vi "HPLC software.vi"() -> ()   [LabVIEW 2014]
panel:
  out "Current Element 3":string
  in  "Baseline":bool
  in  "Lac end":dbl=6.0 format="%.2f"
  in  "Lac start":sgl=5.0 format="%.2f"
  in  "Xyl":dbl=4.0 format="%.2f"
  in  "GluXyl not important":dbl=3.0 format="%.2f"
  in  "Glu":dbl=1.0 format="%.2f"
  out "error out":errorcluster
  in  "Add 6":bool caption="Add"
  in  "Add element 6":string
  in  "Baseline 6":bool
  in  "Reset list 6":bool
  in  "Add 5":bool caption="Add"
  in  "Add element 5":string
  in  "Baseline 5":bool
  in  "Reset list 5":bool
  in  "Add 4":bool caption="Add"
  in  "Add element 4":string
  in  "Baseline 4":bool
  in  "Reset list 4":bool
  out "mean 3":dbl format="%0.2f"
  in  "Baseline 3":bool
  in  "Baseline 2":bool
  in  "Add element 2":string
  in  "Add 2":bool caption="Add"
  in  "Reset list 2":bool
  out "Glu concentration":dbl format="%.4f"
  out "?":cluster{"all rows":dbl[], "all rows":dbl[]}(graph)
  out "Xyl concentration":dbl format="%.4f"
  out "Lac concentration":dbl format="%.4f"
  in  "Glu standard area":dbl=2.0 format="%.2f"
  in  "Xyl standard area":dbl=3.0 format="%.2f"
  out "Glu area":dbl format="%.4f"
  out "Xyl area":dbl format="%.4f"
  in  "Lac standard area":dbl=4.0 format="%.2f"
  out "Lac area":dbl format="%.4f"
  in  "Reset list":bool
  in  "Add":bool
  in  "Add element 1":string
  in  "Path 1":path
  in  "Path 2":path
  in  "Path 4":path
  in  "Path 5":path
  in  "Path 6":path
  out "mean 6":dbl format="%0.2f"
  out "Device 6":cluster{dbl[], dbl[]}(graph)
  out "Current Element 6":string
  out "All samples":i32
  in  "Sample list 6":i32(listbox)
  out "Elapsed Time (s) 6":dbl
  in  "Time Target (s) 6":dbl=1.0
  out "mean 5":dbl format="%0.2f"
  out "Device 5":cluster{dbl[], dbl[]}(graph)
  out "Current Element 5":string
  out "All samples":i32
  in  "Sample list 5":i32(listbox)
  out "Elapsed Time (s) 5":dbl
  in  "Time Target (s) 5":dbl=1.0
  out "mean 4":dbl format="%0.2f"
  out "Device 4":cluster{dbl[], dbl[]}(graph)
  out "Current Element 4":string
  out "All samples":i32
  in  "Sample list 4":i32(listbox)
  out "Elapsed Time (s) 4":dbl
  in  "Time Target (s) 4":dbl=1.0
  out "JJ channel 2":cluster{dbl[], dbl[]}(graph)
  out "mean 2":dbl format="%0.2f"
  out "JJ channel 1":cluster{dbl[], dbl[]}(graph)
  out "Current Element 2":string
  out "All samples":i32
  in  "Sample list 2":i32(listbox)
  out "Elapsed Time (s) 2":dbl
  in  "Time Target for last measurement 2":dbl=1.0
  out "mean 1":dbl format="%0.2f"
  in  "VISA Port":refnum<visa-resource-name>
  out "Current Element":string
  out "Sugar column":cluster{dbl[], dbl[]}(graph)
  in  "Sample list":i32(listbox)=-1
  out "All samples":i32
  out "Elapsed Time (s)":dbl
  in  "Time Target (s)":dbl=1.0
  in  "stop":bool
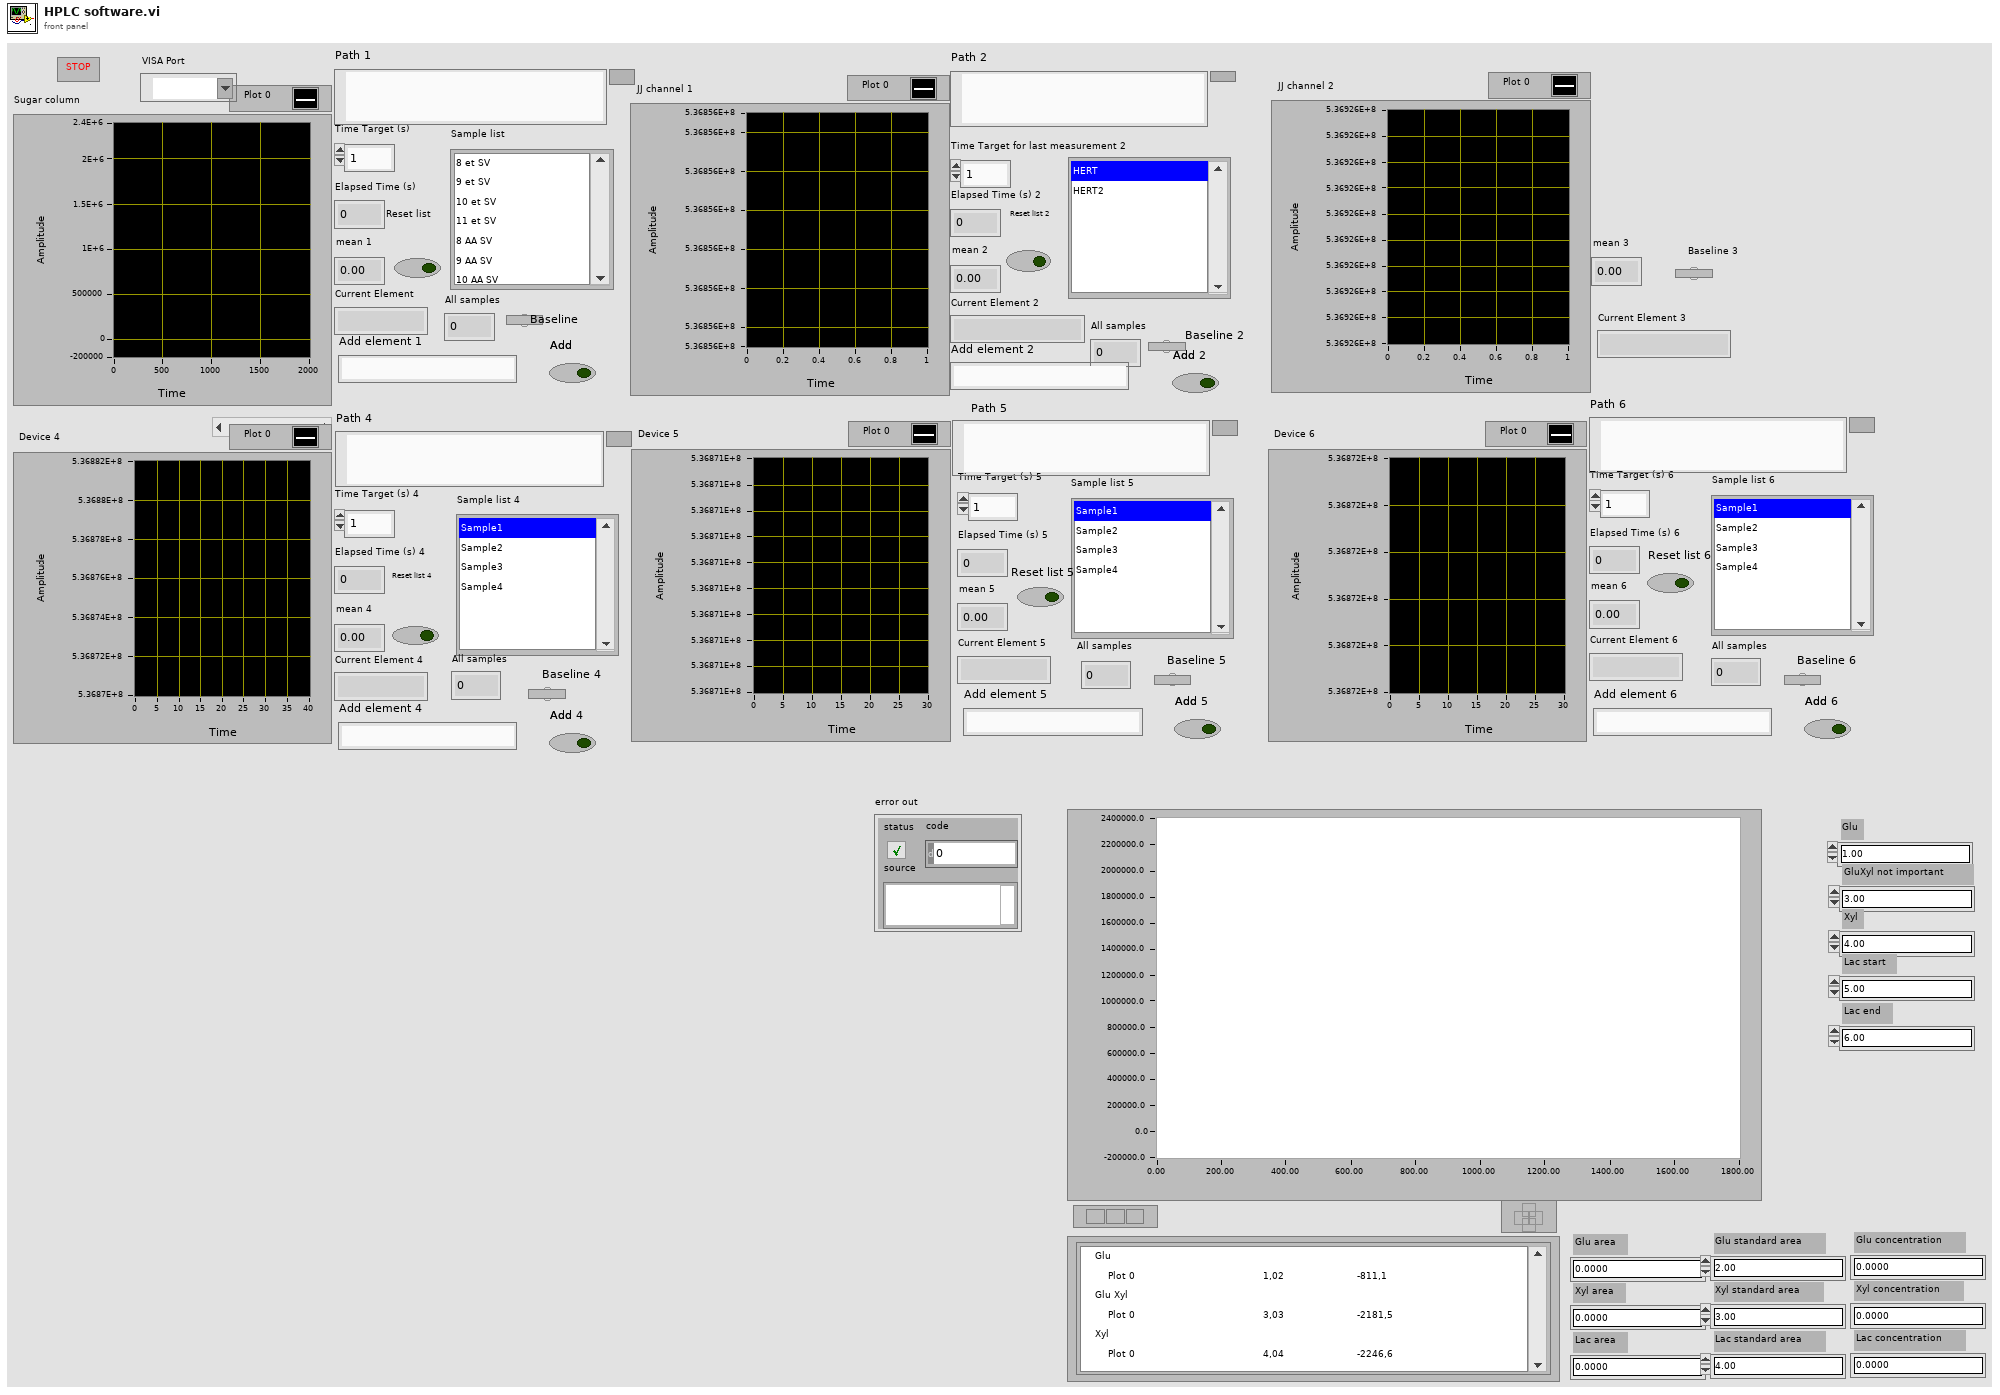
[diagram p1: front panel]
types:
  T1 = cluster{"mean":dbl, "mean":dbl, "mean":dbl, "mean":dbl, "mean":dbl, "mean":dbl}
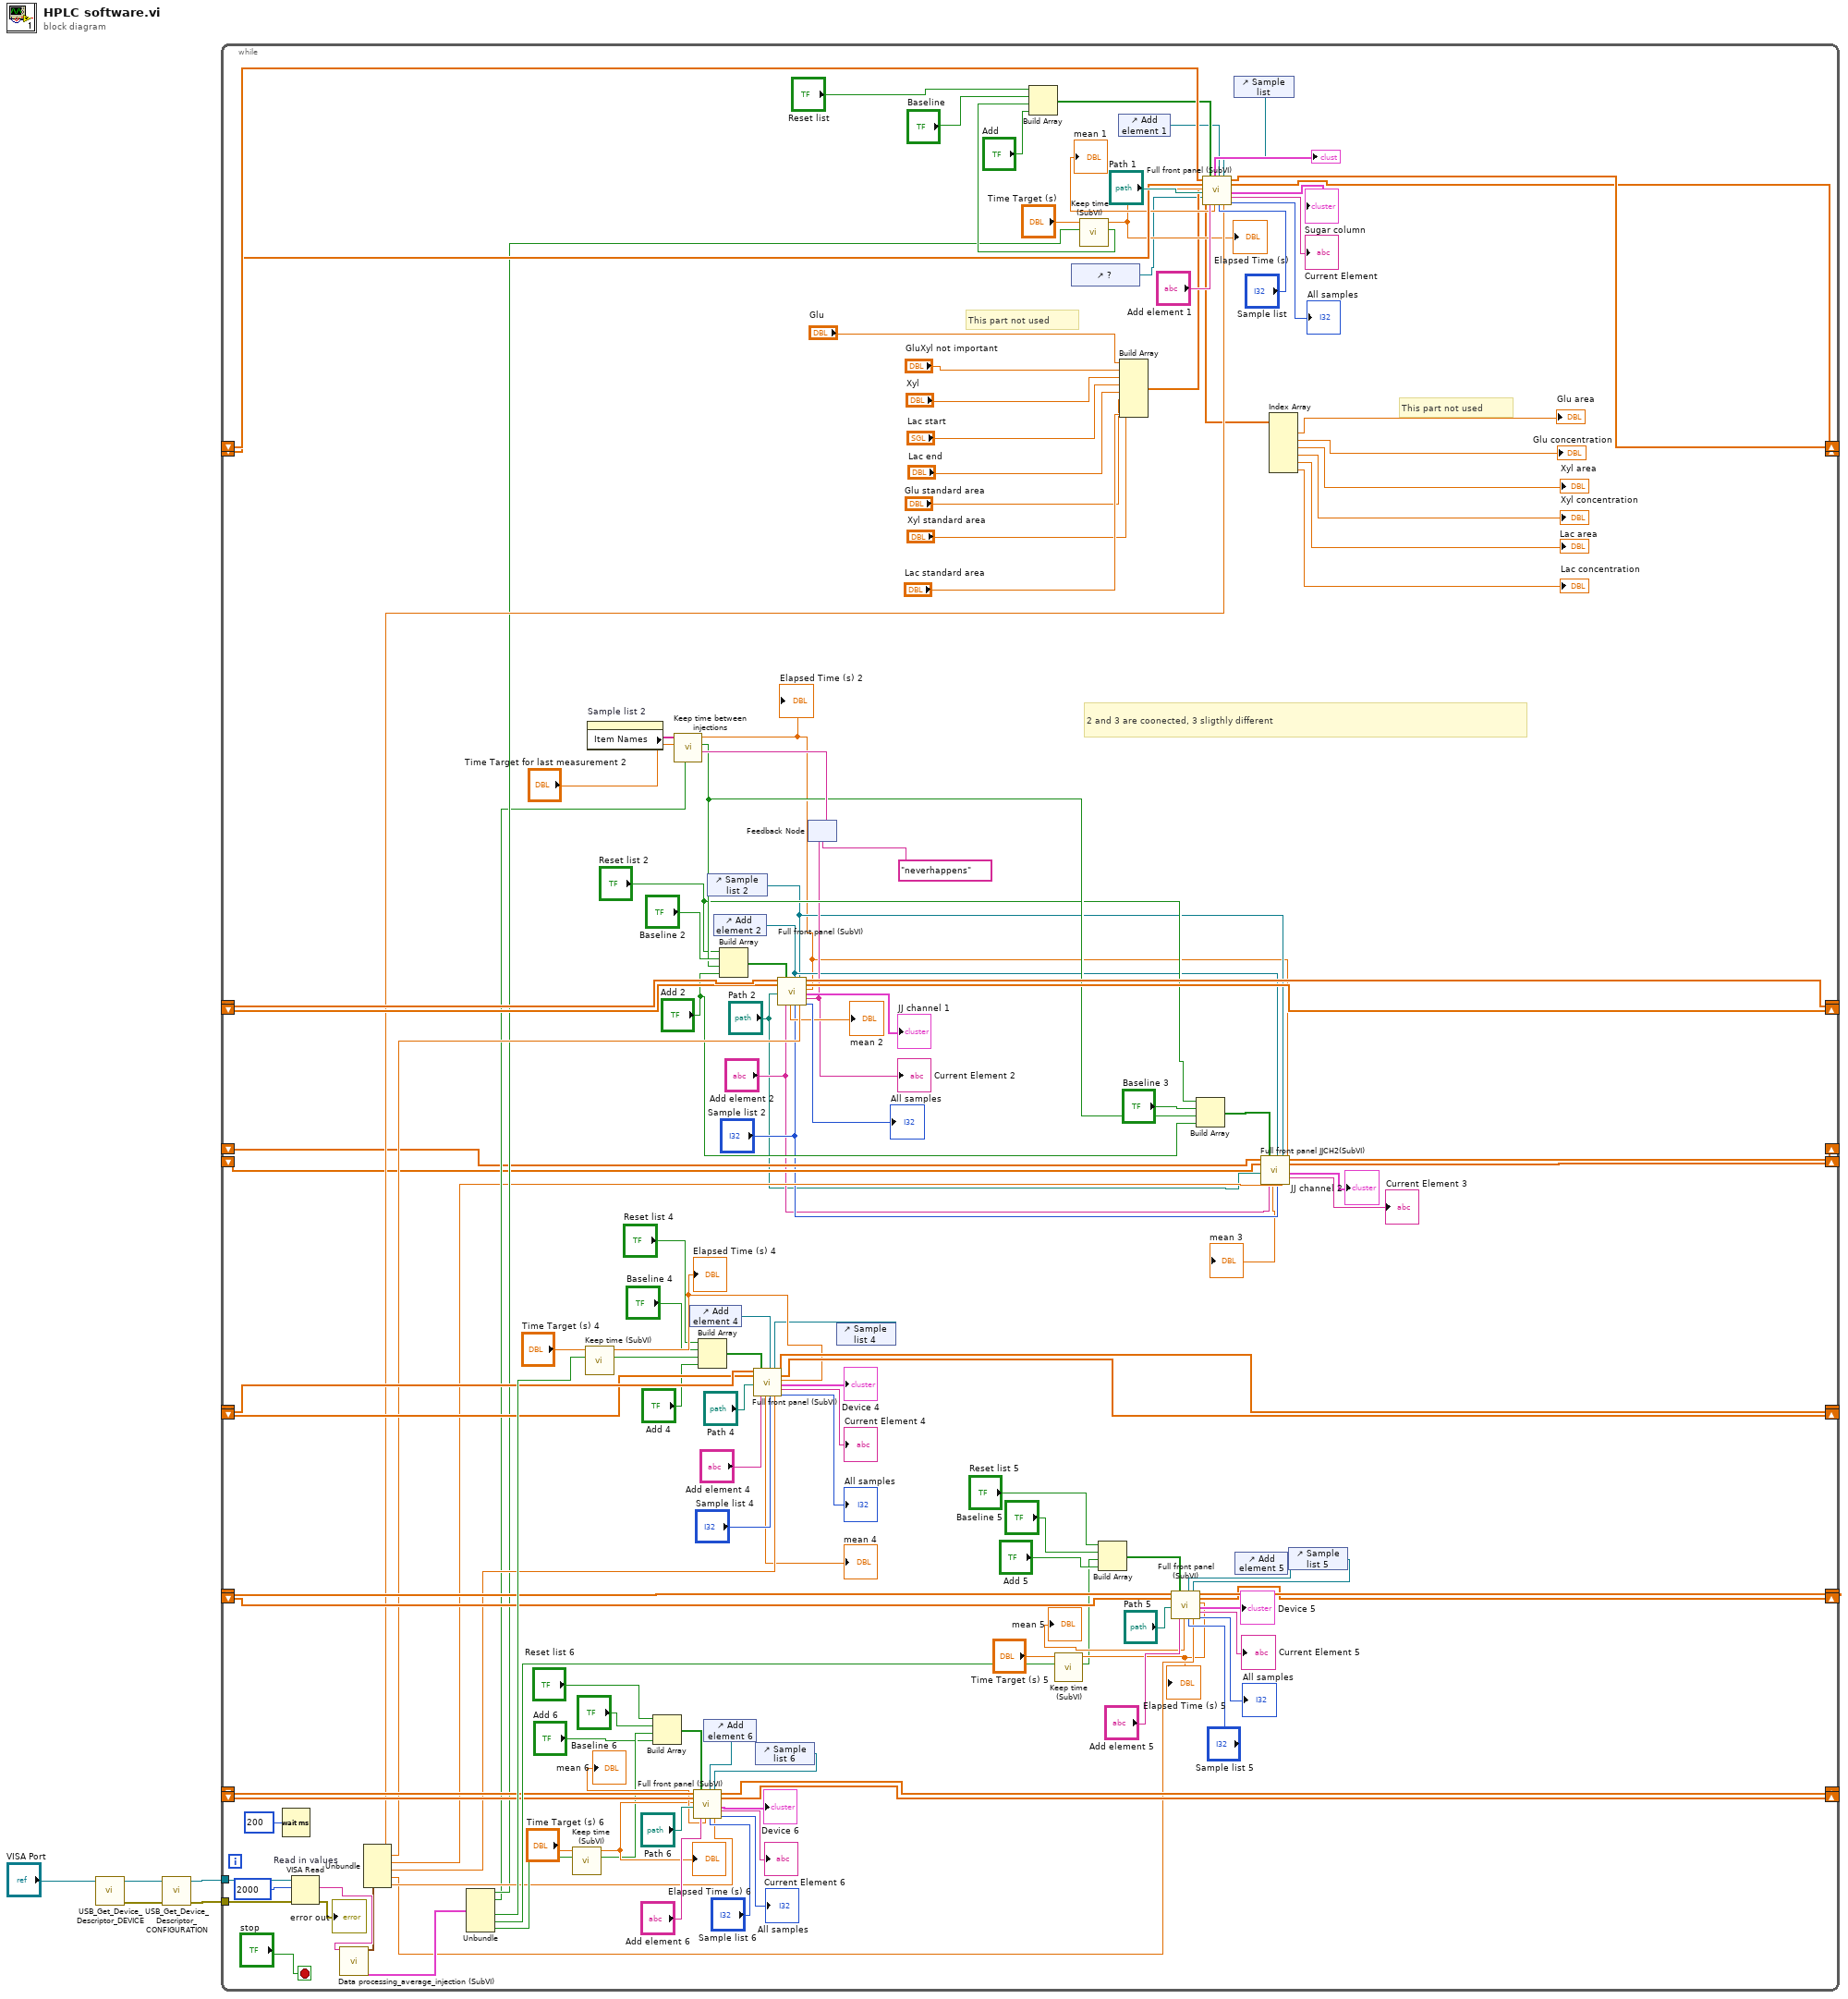
[diagram p0: block diagram]
diagram:
  n1 = call "USB_Get_Device_Descriptor_DEVICE.vi"("VISA resource name"="VISA Port") -> ("error out"=w4:errorcluster, "VISA resource name 2"=w5:refnum<visa-resource-name>)  [unwired: 4 in, 1 out]
  n2 = call "USB_Get_Device_Descriptor_CONFIGURATION.vi"("error out 2"=w4, "VISA resource name"=w5) -> ("error out"=w2:errorcluster, "VISA resource name 2"=w3:refnum<visa-resource-name>)  [unwired: 2 in, 2 out]
  n3 = while {
    shift-right: [w115] -> _
    shift-left: _ -> [w117]
    shift-right: [w114] -> _
    shift-left: _ -> [w116]
    tunnel: w3 -> [w154]
    tunnel: w2 -> [w152]
    shift-right: [w124] -> _
    shift-left: _ -> [w96]
    shift-right: [w125] -> _
    shift-left: _ -> [w97]
    shift-right: [w131] -> _
    shift-left: _ -> [w135]
    shift-right: [w130] -> _
    shift-left: _ -> [w134]
    shift-right: [w15] -> _
    shift-left: _ -> [w17]
    shift-right: [w14] -> _
    shift-left: _ -> [w16]
    shift-right: [w129] -> _
    shift-left: _ -> [w127]
    shift-right: [w128] -> _
    shift-left: _ -> [w126]
    shift-right: [w105] -> _
    shift-left: _ -> [w107]
    shift-right: [w104] -> _
    shift-left: _ -> [w106]
    stop <- "stop" stop-if-true
    # "2 and 3 are coonected, 3 sligthly different"
    # "This part not used"
    # "This part not used"
    n4 = Wait (ms)(milliseconds to wait=u32 200) -> ()  [unwired: 1 out]
    n5 = VISA Read "Read in values"(VISA resource name=w154, byte count=u32 2000, error in (no error)=w152) -> (read buffer=w153:string, error out=→"error out":errorcluster)  [unwired: 2 out]
    n6 = call "Data processing_average_injection (SubVI).vi"("Measurement input"=w153) -> ("output cluster 2"=w146:T1, "output cluster"=w145:cluster{bool, bool, bool, bool, bool, bool})  [unwired: 25 in]
    n7 = Unbundle(w146) -> ("mean"=w95:dbl, "mean"=w89:dbl, "mean"=w10:dbl, "mean"=w92:dbl, "mean"=w93:dbl, "mean"=w94:dbl)
    n8 = Unbundle(w145) -> (w55:bool, w29:bool, w142:bool, w143:bool, w144:bool)  [unwired: 1 out]
    n9 = call "Keep time (SubVI).vi"("Injection"=w144, "Time Target (s)"="Time Target (s) 6") -> ("Measurement running?"=w41:bool, "Elapsed Time (s)"=w81:dbl)  [unwired: 8 in]
    "Elapsed Time (s) 6" <- w81
    n10 = call "Keep time (SubVI).vi"("Injection"=w142, "Time Target (s)"="Time Target (s) 4") -> ("Measurement running?"=w48:bool, "Elapsed Time (s)"=w83:dbl)  [unwired: 8 in]
    "Elapsed Time (s) 4" <- w83
    n11 = property on="Sample list 2" class="LstBox (strict)"() -> ("Item Names"=w28:string[])  [unwired: 2 in, 2 out]
    n12 = Build Array("Reset list 6", "Baseline 6", w41, "Add 6") -> (w39:bool[])
    n13 = control-ref of="Add element 4"() -> (w45:refnum<vi>)
    n14 = Build Array("Reset list 4", "Baseline 4", w48, "Add 4") -> (w46:bool[])
    n15 = control-ref of="Add element 6"() -> (w38:refnum<vi>)
    n16 = control-ref of="Sample list 2"() -> (w18:refnum<vi>)
    n17 = control-ref of="Add element 2"() -> (w19:refnum<vi>)
    n18 = control-ref of="Sample list 6"() -> (w37:refnum<vi>)
    n19 = call "Full front panel (SubVI).vi"("Signal in"=w107, "Time in"=w106, "Path 1"="Path 6", "Boolean"=w39, "Add element 1"="Add element 6", "String"=w38, "Sample list"="Sample list 6", "Sample list 2"=w37, "mean In"=w94, "Elapsed Time (s)"=w81) -> ("Mean"=→"mean 6":dbl, "Signal out"=w105:dbl[], "Time out"=w104:dbl[], "Plot"=→"Device 6":cluster{dbl[], dbl[]}, "Current Element"=→"Current Element 6":string, "All samples"=→"All samples":i32)  [unwired: 2 in, 2 out]
    n20 = feedback #1("neverhappens" ("Current Element")) -> (w27:string)
    n21 = call "Keep time between injections.vi"("Boolean in"=w29, "Current Element"=w27, "Time Target for last measurement in"="Time Target for last measurement 2", "Item Names"=w28) -> ("Boolean out"=w24:bool, "Elapsed Time (s)"=w13:dbl)  [unwired: 6 in]
    "Elapsed Time (s) 2" <- w13
    n22 = Build Array("Reset list 2", "Baseline 2", w24, "Add 2") -> (w52:bool[])
    n23 = call "Full front panel (SubVI).vi"("Signal in"=w135, "Time in"=w134, "Path 1"="Path 2", "Boolean"=w52, "Add element 1"="Add element 2", "String"=w19, "Sample list"="Sample list 2", "Sample list 2"=w18, "mean In"=w89, "Elapsed Time (s)"=w13) -> ("Mean"=→"mean 2":dbl, "Signal out"=w131:dbl[], "Time out"=w130:dbl[], "Plot"=→"JJ channel 1":cluster{dbl[], dbl[]}, "Current Element"=w21:string, "All samples"=→"All samples":i32)  [unwired: 2 in, 2 out]
    "Current Element 2" <- w21
    n24 = feedback-in #1(w21) -> ()
    n25 = control-ref of="Sample list 4"() -> (w44:refnum<vi>)
    n26 = call "Full front panel (SubVI).vi"("Signal in"=w127, "Time in"=w126, "Path 1"="Path 4", "Boolean"=w46, "Add element 1"="Add element 4", "String"=w45, "Sample list"="Sample list 4", "Sample list 2"=w44, "mean In"=w92, "Elapsed Time (s)"=w83) -> ("Mean"=→"mean 4":dbl, "Signal out"=w129:dbl[], "Time out"=w128:dbl[], "Plot"=→"Device 4":cluster{dbl[], dbl[]}, "Current Element"=→"Current Element 4":string, "All samples"=→"All samples":i32)  [unwired: 2 in, 2 out]
    n27 = call "Keep time (SubVI).vi"("Injection"=w143, "Time Target (s)"="Time Target (s) 5") -> ("Measurement running?"=w32:bool, "Elapsed Time (s)"=w82:dbl)  [unwired: 8 in]
    "Elapsed Time (s) 5" <- w82
    n28 = control-ref of="?"() -> (w61:refnum<vi>)
    n29 = call "Keep time (SubVI).vi"("Injection"=w55, "Time Target (s)"="Time Target (s)") -> ("Measurement running?"=w65:bool, "Elapsed Time (s)"=w84:dbl)  [unwired: 8 in]
    "Elapsed Time (s)" <- w84
    n30 = Build Array("Reset list", "Baseline", w65, "Add") -> (w66:bool[])
    n31 = Build Array("Reset list 5", "Baseline 5", w32, "Add 5") -> (w33:bool[])
    n32 = control-ref of="Add element 1"() -> (w62:refnum<vi>)
    n33 = Build Array("Glu", "GluXyl not important", "Xyl", "Lac start", "Lac end", "Glu standard area", "Xyl standard area", "Lac standard area") -> (w80:dbl[])
    n34 = Build Array("Reset list 2", "Baseline 3", w24, "Add 2") -> (w20:bool[])
    n35 = control-ref of="Sample list"() -> (w63:refnum<vi>)
    n36 = call "Full front panel (SubVI).vi"("Signal in"=w97, "Time in"=w96, "Integrate Array"=w80, "Path 1"="Path 1", "XYGraph Refnum"=w61, "Boolean"=w66, "Add element 1"="Add element 1", "String"=w62, "Sample list"="Sample list", "Sample list 2"=w63, "mean In"=w95, "Elapsed Time (s)"=w84) -> ("Concentrations"=w75:dbl[], 8:→"?":cluster{"all rows":dbl[], "all rows":dbl[]}, "Mean"=→"mean 1":dbl, "Signal out"=w125:dbl[], "Time out"=w124:dbl[], "Plot"=→"Sugar column":cluster{dbl[], dbl[]}, "Current Element"=→"Current Element":string, "All samples"=→"All samples":i32)
    n37 = control-ref of="Add element 5"() -> (w31:refnum<vi>)
    n38 = call "Full front panel JJCH2(SubVI).vi"("Signal in"=w17, "Time in"=w16, "Path 1"="Path 2", "Boolean"=w20, "Add element 1"="Add element 2", "String"=w19, "Sample list"="Sample list 2", "Sample list 2"=w18, "mean In"=w10, "Elapsed Time (s)"=w13) -> ("Mean"=→"mean 3":dbl, "Signal out"=w15:dbl[], "Time out"=w14:dbl[], "Plot"=→"JJ channel 2":cluster{dbl[], dbl[]}, "Current Element"=→"Current Element 3":string)  [unwired: 2 in, 3 out]
    n39 = Index Array(array=w75) -> (element #1=→"Glu area":dbl, element #2=→"Glu concentration":dbl, element #3=→"Xyl area":dbl, element #4=→"Xyl concentration":dbl, element #5=→"Lac area":dbl, element #6=→"Lac concentration":dbl)  [unwired: 6 in]
    n40 = control-ref of="Sample list 5"() -> (w30:refnum<vi>)
    n41 = call "Full front panel (SubVI).vi"("Signal in"=w117, "Time in"=w116, "Path 1"="Path 5", "Boolean"=w33, "Add element 1"="Add element 5", "String"=w31, "Sample list"="Sample list 5", "Sample list 2"=w30, "mean In"=w93, "Elapsed Time (s)"=w82) -> ("Mean"=→"mean 5":dbl, "Signal out"=w115:dbl[], "Time out"=w114:dbl[], "Plot"=→"Device 5":cluster{dbl[], dbl[]}, "Current Element"=→"Current Element 5":string, "All samples"=→"All samples":i32)  [unwired: 2 in, 2 out]
  }
